vi "FTW-Panel-FrontPanel-SetCursor.vi"(8 "error in":errorcluster, 10 "Cursor":enum32{"Default", "Busy", "Unset Busy", "Link"}(ring), 11 "VI Ref":refnum<vi>) -> (0 "error out":errorcluster, 3 "VI Ref out":refnum<vi>)   [LabVIEW 2015]
uses:
  error/FTW-ERR-CallChain.vi
  string/FTW-STR-ReplaceWhitespace.vi
  string/FTW-STR-Array-Delimit.vi
panel:
  # "Inputs"
  # "Outputs"
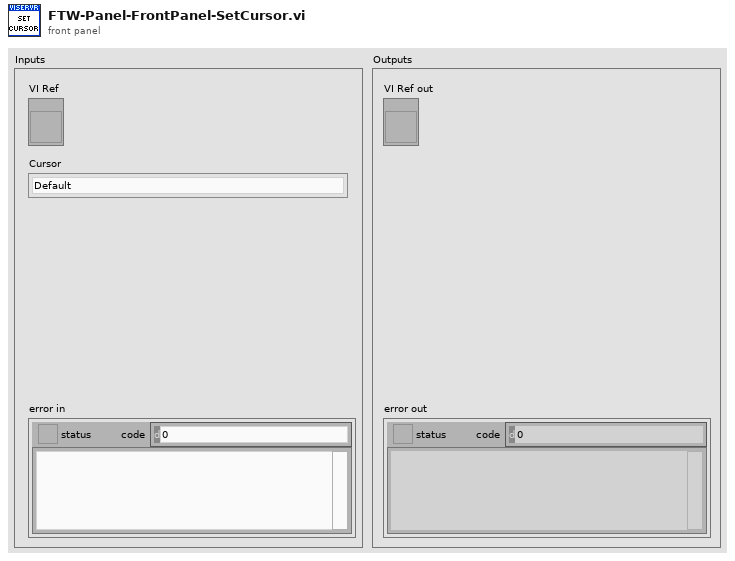
[diagram p1: front panel]
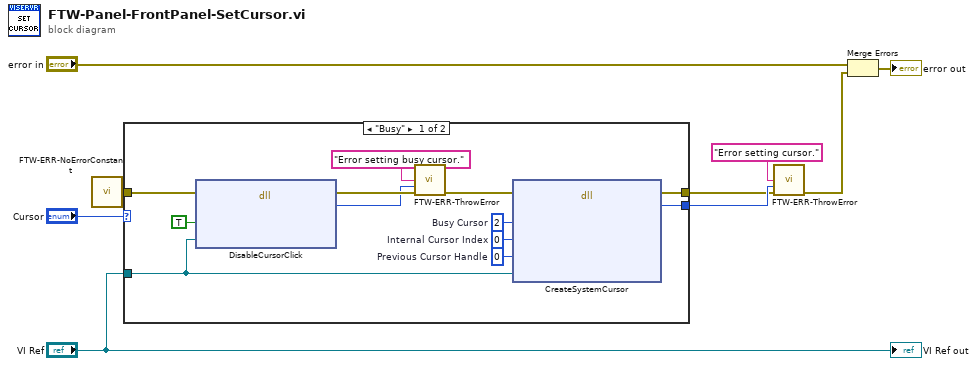
[diagram p0: block diagram]
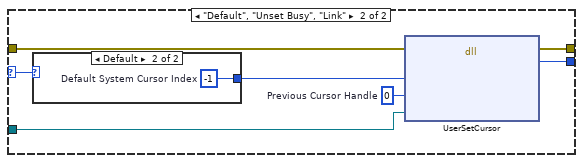
[diagram p2: hidden frame]
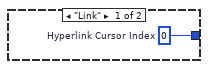
[diagram p3: hidden frame]
diagram:
  n1 = call "FTW-ERR-NoErrorConstant.vi"() -> ("no error"=w1:errorcluster)
  n2 = case shown="\"Busy\"" "Cursor" {
    selector: "Cursor" -> [_ w24]
    tunnel: "VI Ref" -> [w11 w28]
    tunnel: [w12 w27] -> w7
    tunnel: [w13 w26] -> w6
    tunnel: w1 -> [w10 w22]
    frame "Busy" {
      w14 = 0  # Internal Cursor Index
      w15 = 0  # Previous Cursor Handle
      w16 = 2  # Busy Cursor
      n3 = dll-call lib="LabVIEW" fn="DisableCursorClick"(error in=w10, "Disable Click?"=TRUE, "VI Ref"=w11) -> (error out=w20:errorcluster, "Return"=w19:i32)  [unwired: 4 in, 1 out]
      n4 = call "FTW-ERR-ThrowError.vi"("Error Message"="Error setting busy cursor.", "Error Code"=w19, "error in"=w20) -> ("error out"=w17:errorcluster)  [unwired: 12 in]
      n5 = dll-call lib="LabVIEW" fn="CreateSystemCursor"(error in=w17, "Cursor Index"=w16, "Internal Cursor Index"=w14, "Previous Cursor Handle"=w15, "VI Ref"=w11) -> (error out=w13:errorcluster, "Return"=w12:i32)  [unwired: 6 in, 1 out]
    }
    frame "Default", "Unset Busy", "Link" {
      w25 = 0  # Previous Cursor Handle
      n6 = case shown="Default" w24 {
        tunnel: [w29 w30] -> w23
        frame "Link" {
          w29 = 0  # Hyperlink Cursor Index
        }
        frame Default {
          w30 = -1  # Default System Cursor Index
        }
      }
      n7 = dll-call lib="LabVIEW" fn="UserSetCursor"(error in=w22, "Internal Cursor Index"=w23, "Previous Cursor Handle"=w25, "VI Ref"=w28) -> (error out=w26:errorcluster, "Return"=w27:i32)  [unwired: 5 in, 1 out]
    }
  }
  n8 = call "FTW-ERR-ThrowError.vi"("Error Message"="Error setting cursor.", "Error Code"=w7, "error in"=w6) -> ("error out"=w2:errorcluster)  [unwired: 12 in]
  n9 = Merge Errors("error in", w2) -> (→"error out":errorcluster)
  "VI Ref out" <- "VI Ref"
